vi "Scripted Autonomous.vi"   [LabVIEW 2016]
uses:
  Common Code/Drivetrain Mode.ctl
  Common Code/Unload Mode.ctl
  Common Code/Utilities/Change Detect Int.vi
  Robot Global Data.vi
types:
  T1 = typedef "Drivetrain Mode.ctl" = enum16{"Manual", "Gyro Steer", "Distance Drive", "Translate Drive", "Goal Vision Align", "PID Drive"}
  T2 = typedef "Unload Mode.ctl" = enum16{"None", "Close", "Far"}
  T3 = typedef "Dashboard Control Data.ctl" = cluster{"Drivetrain Settings":T4, "Intake Presets ":T7, "Shooter Presets":T8, "Vision Target Packet":T9, "Auton Presets":cluster{"Start Position":dbl}, "Drivetrain Encoder Values":T10, "Drivetrain Encoder Settings":cluster{"Left Tick Constant":dbl, "Right Tick Contant":dbl, "Reset Encoders":bool, "Center Tick Constant":dbl}, "Zero Gyro":bool, "Vision Timeout":dbl, "Pressure M":dbl, "Pressure B":dbl, "Auto Agitator":T12, "Climber Settings":T13, "LEDs":T14}
  T4 = typedef "Drivetrain Settings.ctl" = cluster{"Gyro Tolerance":dbl, "Gyro Steer PID Gains":T5, "Y Power Multiplier":dbl, "Turn Power Multiplier":dbl, "Gyro Output":dbl, "Creep Rate":dbl, "Distance Drive PID Gains":T5, "Distance Tolerance":dbl, "Distance Output":dbl, "Strafe Threshold":dbl, "Strafe Correct":bool, "Strafe Tolerance":dbl, "Translate Drive PID Gains":T5, "Strafe Output":dbl, "SC Right":dbl, "SC Left":dbl, "Use Gyro":bool, "Constant Power":bool, "Strafe Power":dbl, "Input Modifier":T6, "SCR Delay":dbl, "SCL Delay":dbl}
  T5 = typedef "PID Gains.ctl" = cluster{"proportional gain (Kc)":dbl, "integral time (Ti, min)":dbl, "derivative time (Td, min)":dbl}
  T6 = typedef "Input Modifier.ctl" = enum16{"None", "Square", "Cube"}
  T7 = typedef "Intake Presets.ctl" = cluster{"Intake Speed ":dbl, "Outake Speed":dbl, "Current Trip Delay":dbl, "Max Current":dbl, "Gear Outtake Motor Delay":dbl, "Gear Intake Motor Delay":dbl, "Gear Intake Pull Up Speed":dbl, "Pusher Delay":dbl, "Release Delay":dbl, "Close Release Delay":dbl}
  T8 = typedef "Shooter Presets.ctl" = cluster{"Key Shot":cluster{"RPM ":dbl, "Hood?":bool}, "Distance Shot":cluster{"RPM":dbl, "Hood?":bool}, "RPM Tolerance":dbl, "Unstuck Delay Time ":dbl, "Initial RPM Increase":dbl, "Warmup Delay":dbl, "Faster Time":dbl, "Shooter PID Gains":cluster{"P":dbl, "I":dbl, "D":dbl, "FF":dbl, "Ramp Rate":dbl, "I Zone":dbl}, "Unstuck Trigger Power":dbl, "Trigger Power":dbl, "Unstuck RPM":dbl, "Agitator Active Power":dbl, "Agitator Idle Power":dbl, "RPM Tuning Range":dbl, "RPM M Tuning Range":dbl}
  T9 = typedef "Vision Target Packet.ctl" = cluster{"Robot Center":dbl, "Center X":dbl, "Center Y":dbl, "Angle":dbl, "Distance":dbl, "Found Target?":bool}
  T10 = typedef "Drivetrain Encoder Values.ctl" = cluster{"Left Encoder":T11, "Center Encoder":T11, "Right Encoder":T11}
  T11 = typedef "Encoder Values.ctl" = cluster{"Distance":dbl, "Speed":dbl, "Tick":dbl}
  T12 = typedef "Auto Agitator Settings.ctl" = cluster{"Enable Auto Agitation":bool, "Continuous Stir":bool, "Continuous Intake":bool, "Alternate In/Outtake":bool, "Wing Delay":dbl, "Stir Delay":dbl, "Intake Delay":dbl, "Wing On Time":dbl, "Wing Off Time":dbl, "Stir On Time":dbl, "Stir Off Time":dbl, "Intake On Time":dbl, "Intake Off Time":dbl, "Stir Power":dbl, "Intake Power":dbl, "Outtake Power":dbl, "Intake Run Time":dbl, "Outtake Run Time":dbl, "Wing$":bool, "Intake":bool, "Stirrer":bool}
  T13 = typedef "Climber Settings.ctl" = cluster{"Climber Power":dbl, "Max Current":dbl, "Avoid Current Trip?":bool}
  T14 = typedef "LED Global Data.ctl" = cluster{"Back":cluster{"Default":string, "Traction":string, "Gear Ready Close":string, "Break On":string, "Gear Loaded":string, "Climb":string, "Gear Ready Far":string, "Unload Gear":string}, "Front":cluster{"Default":string, "Traction":string, "Gear Ready Close":string, "Break On":string, "Gear Loaded":string, "Climb":string, "Gear Ready Far":string, "Unload Gear":string}, "LEDOnTime":dbl, "LEDOffTime":dbl}
  T15 = typedef "Auton Command Cluster.ctl" = cluster{"commandID":dbl, "maxTime":dbl, "distanceTarget":dbl, "headingTarget":dbl, "translationTarget":dbl, "ySpeed":dbl, "xSpeed":dbl, "zSpeed":dbl, "async":dbl, "shotType":dbl, "shootCommand":dbl, "rollerPower":dbl, "fillHopper?":dbl, "zeroGyro":dbl, "openGear":dbl, "traction?":dbl}
  T16 = typedef "Drivetrain Status Cluster.ctl" = cluster{"Drivetrain Mode":enum16{"Manual", "Gyro Steer"}, "Y (Throttle)":dbl, "X (Steer)":dbl, "Z (Strafe)":dbl, "Heading Target":dbl, "Center Piston Down?":bool, "Traction?":bool, "Gyro Steer Finished?":bool, "Distance Drive Finished?":bool, "Gyro":dbl, "Distance Target":dbl, "Y Max Output":dbl, "Y Min Output":dbl, "X Max Output":dbl, "X Min Output":dbl, "Z Max Output":dbl, "Z Min Output":dbl, "Translation Target":dbl, "Translation Drive Finished?":bool, "PID Auto Drive Finished?":bool, "Brake?":bool, "Vision Aligned?":bool, "Creep Mode Engaged?":bool}
  T17 = typedef "Drivetrain Command Cluster.ctl" = cluster{"Drivetrain Mode":T1, "Heading Target":dbl, "Turn Power":dbl, "Y Power":dbl, "Center Piston Down?":bool, "Traction?":bool, "Strafe Power":dbl, "Zero Gyro":bool, "Distance Target":dbl, "Strafe Correct":bool, "Y Max Output":dbl, "Y Min Output":dbl, "X Max Output":dbl, "X Min Output":dbl, "Z Max Output":dbl, "Z Min Output":dbl, "Z Target":dbl, "Brake?":bool}
  T18 = typedef "Intake Control Cluster.ctl" = cluster{"Intake Mode":T19, "Intake Auto Command":T20, "Intake Current Trip State":T21, "Flap Open? / Confirm Outtake?":bool, "Engage traction for gear load?":bool, "Wings open?":bool, "Manual Intake Power":dbl, "Outtake?":bool, "Unload State":T22, "Load State":T23, "Unload Mode":T2}
  T19 = typedef "Intake Modes.ctl" = enum16{"Manual", "Auto"}
  T20 = typedef "Intake Auto States.ctl" = enum16{"Outtake", "Idle", "Intake", "Intake Pull Up"}
  T21 = typedef "Intake Trip States.ctl" = enum16{"Normal", "Backward Tripped", "Forward Tripped"}
  T22 = typedef "Outtake State.ctl" = enum16{"Idle", "Start", "Doors Open", "Push Out"}
  T23 = typedef "Load State.ctl" = enum16{"Idle", "Open Flap", "Ready Close", "Ready Far"}
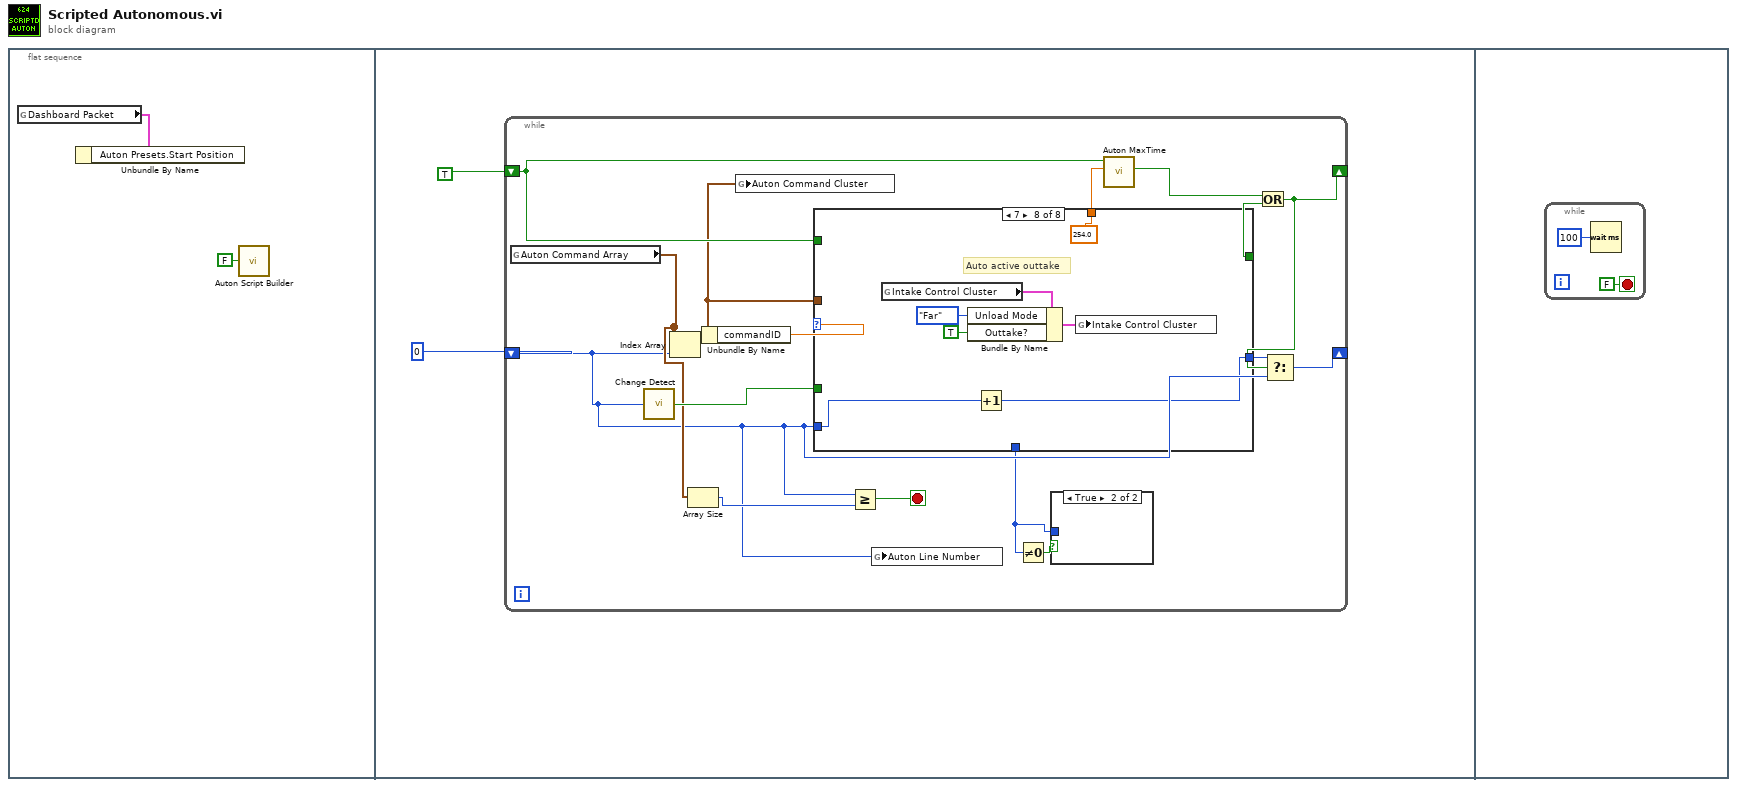
[diagram p0: block diagram]
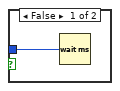
[diagram p2: hidden frame]
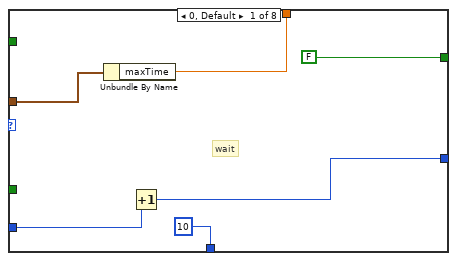
[diagram p3: hidden frame]
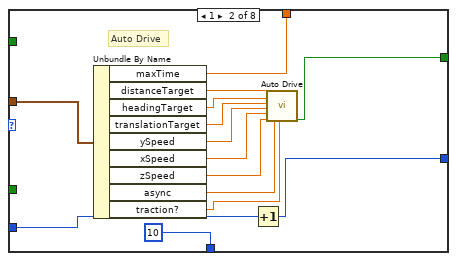
[diagram p4: hidden frame]
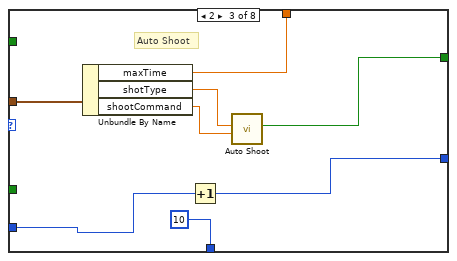
[diagram p5: hidden frame]
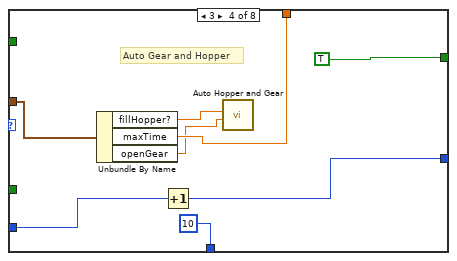
[diagram p6: hidden frame]
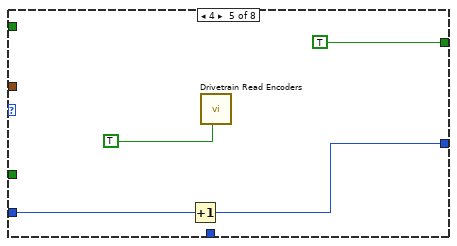
[diagram p7: hidden frame]
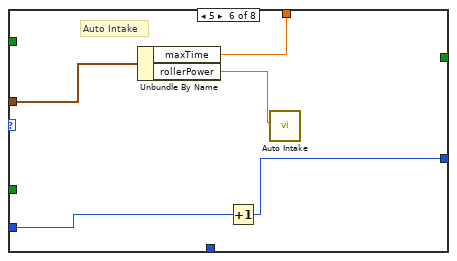
[diagram p8: hidden frame]
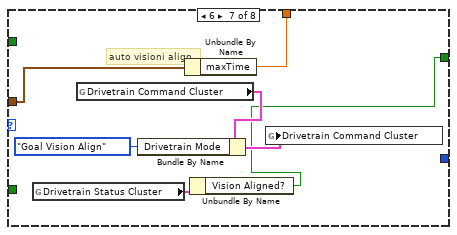
[diagram p9: hidden frame]
diagram:
  n1 = flat-sequence {
    frame #0 {
      n2 = global read "Robot Global Data.vi" "Dashboard Packet"() -> (w1:T3)
      n3 = Unbundle By Name(w1) -> ()  [unwired: 1 out]
      n4 = call "Auton Script Builder.vi"("Export?"=FALSE) -> ()  [unwired: 10 in, 1 out]
    }
    frame #1 {
      n5 = while {
        shift-right: [w12] -> _
        shift-left: TRUE -> [w15]
        shift-right: [w9] -> _
        shift-left: 0 -> [w11]
        stop <- w17 stop-if-true
        n6 = global read "Robot Global Data.vi" "Auton Command Array"() -> (w18:T15[])
        n7 = call-poly "Change Detect.vi"("In"=w11) -> ("Changed?"=w20:bool)
        n8 = Index Array(array=w18, index=w11) -> (element=w5:T15)
        n9 = Array Size(array=w18) -> (size(s)=w16:i32)
        n10 = Unbundle By Name(w5) -> ("commandID"=w19:dbl)
        n11 = global write "Robot Global Data.vi" "Auton Command Cluster"(w5) -> ()
        n12 = case shown="7" w19 {
          tunnel: w20 -> [_ _ _ _ _ _ _ _]
          tunnel: w5 -> [w26 w41 w49 w57 _ w66 w70 _]
          tunnel: w11 -> [w24 w34 w46 w55 w61 w64 _ w80]
          tunnel: w15 -> [_ _ _ _ _ _ _ _]
          tunnel: [FALSE w35 w42 TRUE TRUE ("Finished?") _ w67 _] -> w14
          tunnel: [w23 w33 w45 w54 w60 w63 _ w79] -> w10
          tunnel: [10 10 10 10 _ _ _ _] -> w8
          tunnel: [w25 w32 w48 w56 _ w65 w69 254.0 ("maxTime")] -> w6
          frame 0, Default {
            # "wait"
            n13 = Unbundle By Name(w26) -> ("maxTime"=w25:dbl)
            n14 = Increment(x=w24) -> (x+1=w23:i32)
          }
          frame 1 {
            # "Auto Drive"
            n15 = Unbundle By Name(w41) -> ("maxTime"=w32:dbl, "distanceTarget"=w40:dbl, "headingTarget"=w30:dbl, "translationTarget"=w39:dbl, "ySpeed"=w38:dbl, "xSpeed"=w29:dbl, "zSpeed"=w37:dbl, "async"=w36:dbl, "traction?"=w28:dbl)
            n16 = Increment(x=w34) -> (x+1=w33:i32)
            n17 = call "Auto Drive.vi"("Distance Target"=w40, "Heading Target"=w30, "Strafe Target"=w39, "Y Speed"=w38, "X Speed"=w29, "Z Speed"=w37, "Async?"=w36, "Traction?"=w28) -> ("Finished?"=w35:bool)  [unwired: 11 in]
          }
          frame 2 {
            # "Auto Shoot"
            n18 = Unbundle By Name(w49) -> ("maxTime"=w48:dbl, "shotType"=w44:dbl, "shootCommand"=w43:dbl)
            n19 = Increment(x=w46) -> (x+1=w45:i32)
            n20 = call "Auto Shoot.vi"("Shoot Command"=w43, "Shot Type"=w44) -> ("finished?"=w42:bool)  [unwired: 9 in]
          }
          frame 3 {
            # "Auto Gear and Hopper"
            n21 = Unbundle By Name(w57) -> ("fillHopper?"=w50:dbl, "maxTime"=w56:dbl, "openGear"=w51:dbl)
            n22 = Increment(x=w55) -> (x+1=w54:i32)
            n23 = call "Auto Hopper and Gear.vi"("openGear"=w51, "Fill Hopper?"=w50) -> ()  [unwired: 10 in]
          }
          frame 4 {
            n24 = Increment(x=w61) -> (x+1=w60:i32)
            n25 = call "Drivetrain Read Encoders.vi"("Reset Encoders"=TRUE) -> ()  [unwired: 10 in, 1 out]
          }
          frame 5 {
            # "Auto Intake"
            n26 = Unbundle By Name(w66) -> ("maxTime"=w65:dbl, "rollerPower"=w62:dbl)
            n27 = Increment(x=w64) -> (x+1=w63:i32)
            n28 = call "Auto Intake.vi"("rollerPower"=w62) -> ()  [unwired: 11 in]
          }
          frame 6 {
            # "auto visioni align"
            n29 = global read "Robot Global Data.vi" "Drivetrain Status Cluster"() -> (w68:T16)
            n30 = global read "Robot Global Data.vi" "Drivetrain Command Cluster"() -> (w73:T17)
            n31 = Bundle By Name(cluster=w73, "Drivetrain Mode"=Drivetrain_Mode."Goal Vision Align") -> (w72:T17)
            n32 = Unbundle By Name(w70) -> ("maxTime"=w69:dbl)
            n33 = Unbundle By Name(w68) -> ("Vision Aligned?"=w67:bool)
            n34 = global write "Robot Global Data.vi" "Drivetrain Command Cluster"(w72) -> ()
          }
          frame 7 {
            # "Auto active outtake"
            n35 = global read "Robot Global Data.vi" "Intake Control Cluster"() -> (w78:T18)
            n36 = Bundle By Name(cluster=w78, "Unload Mode"=Unload_Mode."Far", "Outtake?"=TRUE) -> (w77:T18)
            n37 = Increment(x=w80) -> (x+1=w79:i32)
            n38 = global write "Robot Global Data.vi" "Intake Control Cluster"(w77) -> ()
          }
        }
        n39 = Greater Or Equal?(x=w11, y=w16) -> (x >= y?=w17:bool)
        n40 = global write "Robot Global Data.vi" "Auton Line Number"(w11) -> ()
        n41 = Not Equal To 0?(x=w8) -> (x != 0?=w7:bool)
        n42 = case shown="True" w7 {
          tunnel: w8 -> [w21 _]
          frame False {
            n43 = Wait (ms)(milliseconds to wait=w21) -> ()  [unwired: 1 out]
          }
          frame True {
          }
        }
        n44 = call "Auton MaxTime.vi"("MaxTime"=w6, "Reset?"=w15) -> ("Finished?"=w13:bool)  [unwired: 9 in]
        n45 = Or(x=w13, y=w14) -> (x .or. y?=w12:bool)
        n46 = Select(t=w10, s=w12, f=w11) -> (s? t:f=w9:i32)
      }
    }
    frame #2 {
      n47 = while {
        stop <- FALSE stop-if-true
        n48 = Wait (ms)(milliseconds to wait=u32 100) -> ()  [unwired: 1 out]
      }
    }
  }
